vi "mxwScript_Cmnd2Str_linkToPaneArray.vi"(8 "error in (no error)":errorcluster, 11 "data":variant) -> (0 "error out":errorcluster, 3 "outputString":string)   [LabVIEW 2020]
uses:
  codeGenAPISupport.llb/cgAPI_mxwScript_LinkToArrayOnPaneInfo.ctl
  codeGenAPISupport.llb/cgAPI_mxwScript_ConnPaneConnectionType.ctl
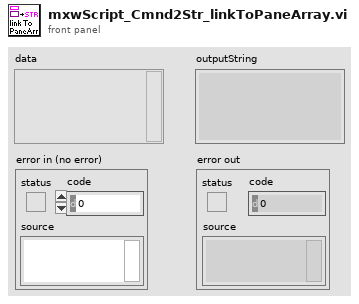
[diagram p1: front panel]
types:
  T1 = typedef "cgAPI_mxwScript_LinkToArrayOnPaneInfo.ctl" = cluster{"controlName":string, "controlTemplateIndex":i32, "paneIndex":i32, "finalName":string, "arrayName":string, "connection type":T2}
  T2 = typedef "cgAPI_mxwScript_ConnPaneConnectionType.ctl" = enum16{"Invalid Wire Rule", "Required", "Recommended", "Optional", "Dynamic Dispatch"}
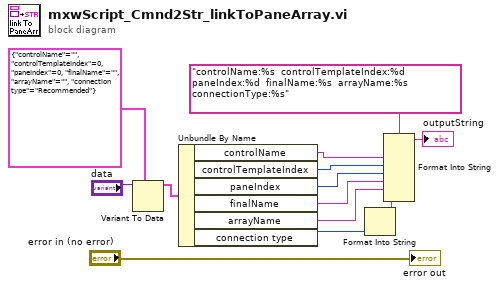
[diagram p0: block diagram]
diagram:
  n1 = Variant To Data(type=T1 {"controlName"="", "controlTemplateIndex"=0, "paneIndex"=0, "finalName"="", "arrayName"="", "connection type"=enum."Recommended"} ("linkToClusterOnPaneInfo"), Variant="data") -> (data=w12:T1)  [unwired: 1 in, 1 out]
  n2 = Unbundle By Name(w12) -> ("controlName"=w8:string, "controlTemplateIndex"=w6:i32, "paneIndex"=w7:i32, "finalName"=w5:string, "arrayName"=w1:string, "connection type"=w4:T2)
  n3 = Format Into String(w4) -> (resulting string=w3:string)  [unwired: 3 in, 1 out]
  n4 = Format Into String(format string="controlName:%s  controlTemplateIndex:%d  paneIndex:%d  finalName:%s  arrayName:%s  connectionType:%s", w8, w6, w7, w5, w1, w3) -> (resulting string=→"outputString":string)  [unwired: 2 in, 1 out]
  "error out" <- "error in (no error)"
